vi "Golander pump(mL per s, mL per rev) old.vi"(4 "State":i16, 5 "Time":dbl format="%.2f", 6 "Sensor Values":dbl[](array[numeric]), 7 "Set Points":dbl[](array[numeric])=[12.0, 1.0, 1.0, 1.0]) -> (0 "required data":T4={"Set Point names"=["com port", "pump address", "on state (-1=all, 167= states 1, 6, 7)", "pump (mL/rev)", "flow (mL/s)"], "required number of setpoints"=5, "required number of sensors"=0, "Sensor names"=[]}, 3 "output value":dbl)   [LabVIEW 2019]
uses:
  pump 2 flows.ctl
  Pump updates.ctl
  modbusrtu/MB Serial Master Query Write Multiple Registers (poly).vi
panel:
  in  "delay before write":u32=200
  out "Pump updates":T1[](array[typedef]) {"Update Time" format="%.2f"}
  in  "Pump updates":T1 {"Update Time" format="%.2f"}
  in  "Timeout":u32=240
  in  "write interval (s)":dbl=5.0
  out "pump cmd array":T2[](array[typedef])
  out "output cluster":T3
  in  "Pump cmds":T2
  in  "error in (no error)":errorcluster
  out "VISA out":refnum<visa-resource-name>
  out "error out":errorcluster
  # "failure at 80 ms"
  # "Enter the correct information for this control code in the required data structure below. Then make the current value default by right clicking on the border of the data structure. Select \"data operations\" and then select \"make current value default\". These values will be displayed by process controller."
  # "Mode: RTU\nAddresses: 1-247 (User Defined)\nBaud Rate: 9600\nData Bits: 8\nCRC: Even Parity\nStop Bit: 1"
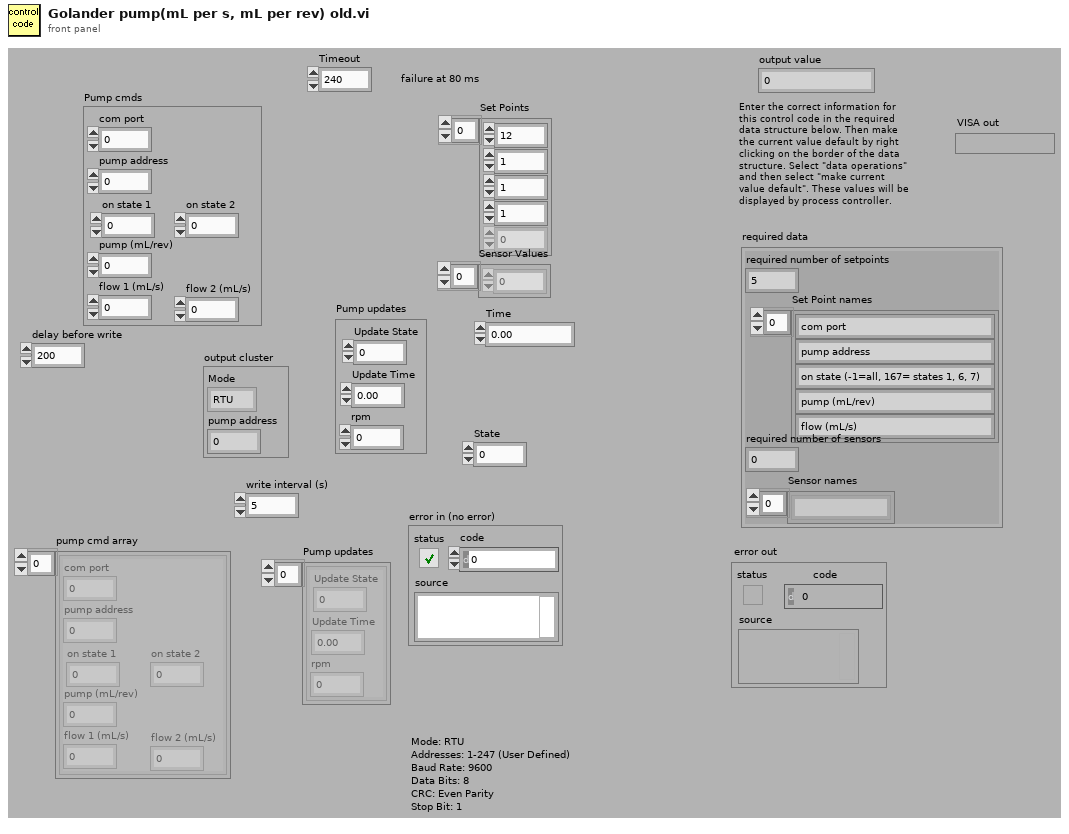
[diagram p1: front panel]
types:
  T1 = typedef "Pump updates.ctl" = cluster{"Update State":i16, "Update Time":dbl, "rpm":dbl}
  T2 = typedef "pump 2 flows.ctl" = cluster{"com port":u8, "pump address":u8, "on state 1":i32, "on state 2":i32, "pump (mL/rev)":dbl, "flow 1 (mL/s)":dbl, "flow 2 (mL/s)":dbl}
  T3 = cluster{"Mode":enum16{"RTU", "ASCII"}, "pump address":u8}
  T4 = cluster{"Set Point names":string[], "required number of setpoints":u8, "required number of sensors":u8, "Sensor names":string[]}
  T5 = cluster{"Set Points[0]":dbl, "Set Points[1]":dbl, "Set Points[2]":dbl, "Set Points[3]":dbl, "Set Points[4]":dbl}
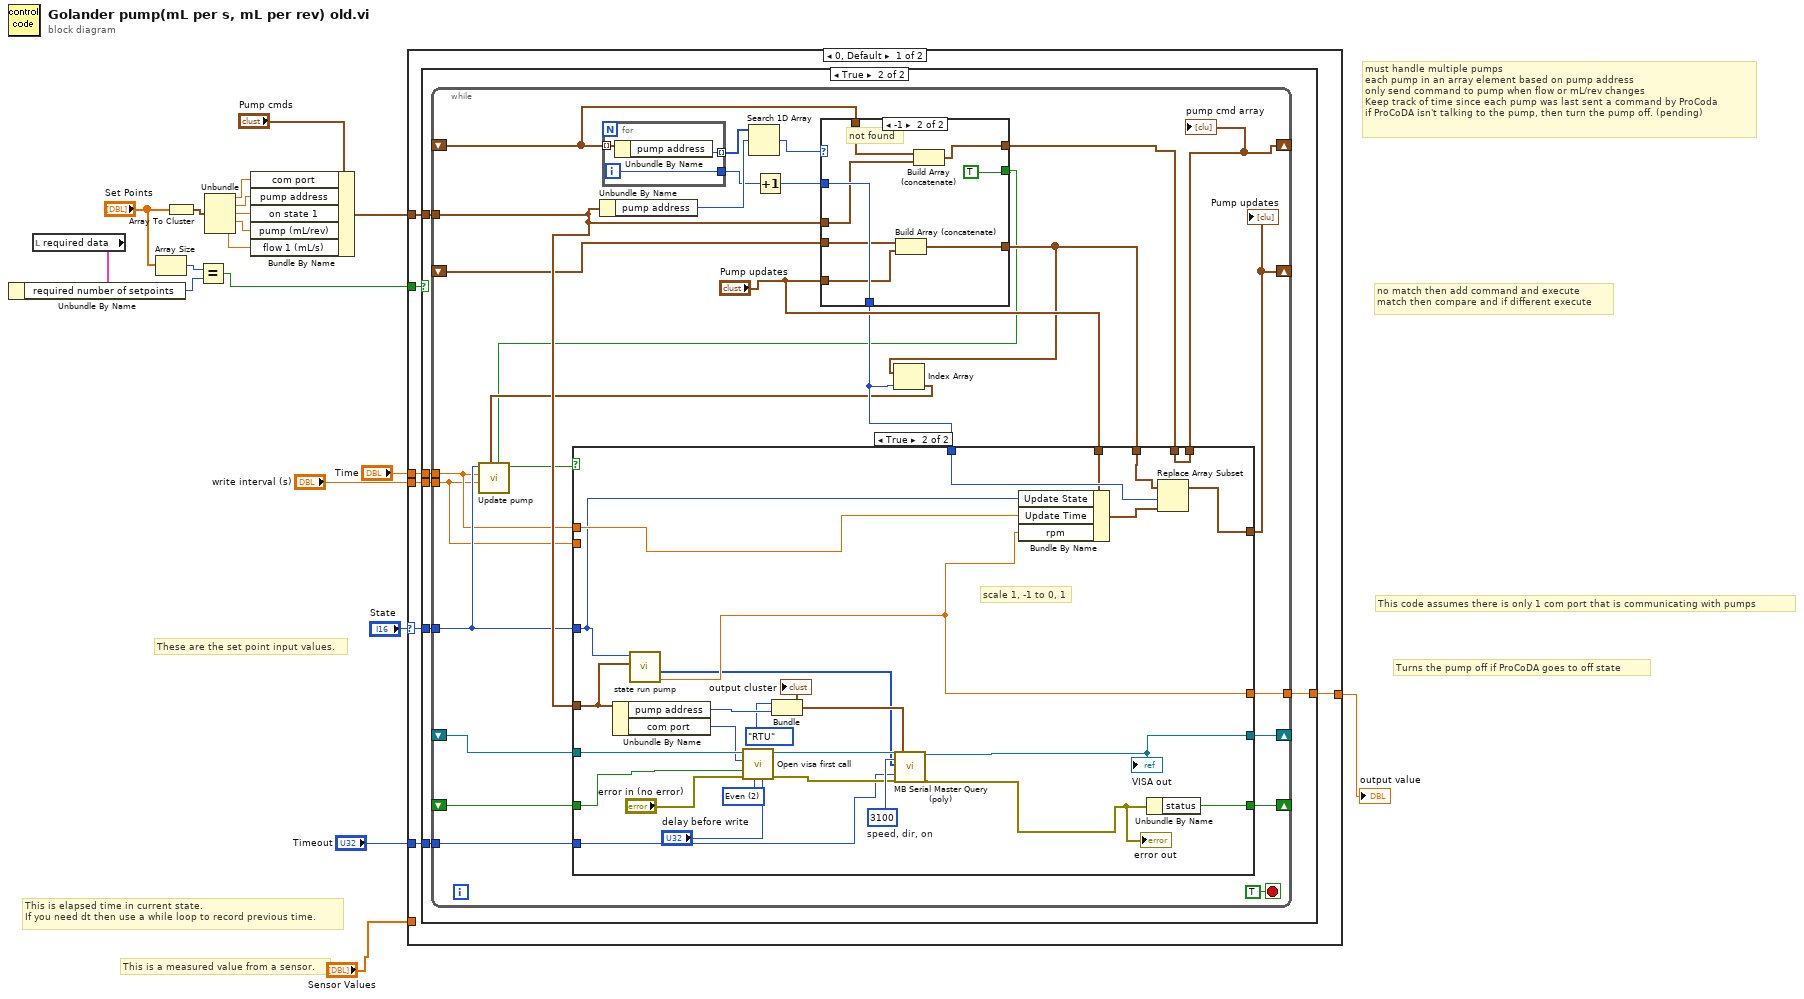
[diagram p0: block diagram]
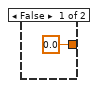
[diagram p2: hidden frame]
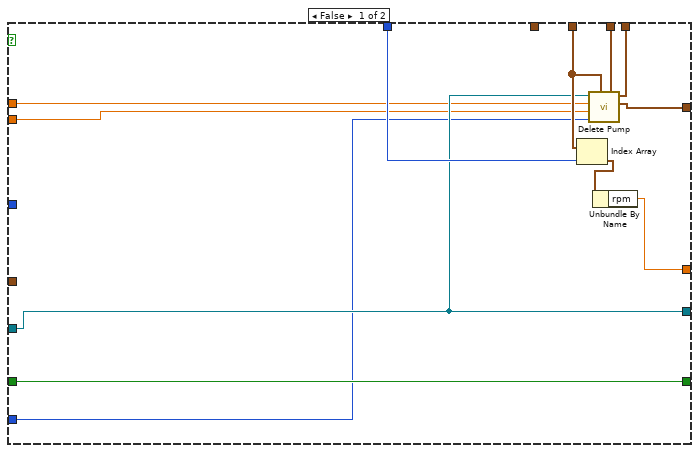
[diagram p3: hidden frame]
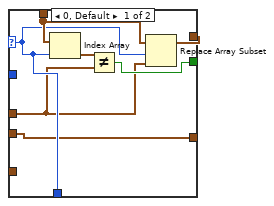
[diagram p4: hidden frame]
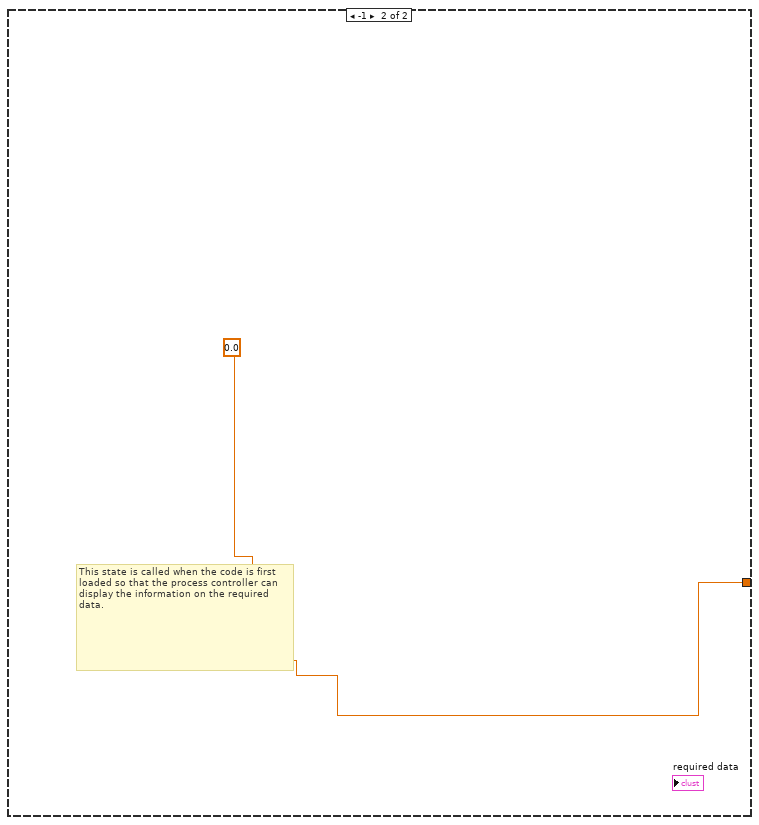
[diagram p5: hidden frame]
diagram:
  # "Turns the pump off if ProCoDA goes to off state"
  # "This code assumes there is only 1 com port that is communicating with pumps"
  # "no match then add command and execute\nmatch then compare and if different execute"
  # "must handle multiple pumps\neach pump in an array element based on pump address\nonly send command to pump when flow or mL/rev changes\nKeep track of time since each pump was last sent a command by ProCoda\nif ProCoDA isn't talking to the pump, then turn the pump off. (pending)"
  # "These are the set point input values."
  # "This is a measured value from a sensor."
  # "This is elapsed time in current state.\nIf you need dt then use a while loop to record previous time."
  n1 = local read "required data"() -> (w3:T4)
  n2 = Unbundle By Name(w3) -> ("required number of setpoints"=w2:u8)
  n3 = Array Size(array="Set Points") -> (size(s)=w5:i32)
  n4 = Array To Cluster(array="Set Points") -> (cluster=w16:T5)
  n5 = Equal?(x=w5, y=w2) -> (x = y?=w1:bool)
  n6 = Unbundle(w16) -> ("Set Points[0]"=w13:dbl, "Set Points[1]"=w17:dbl, "Set Points[2]"=w8:dbl, "Set Points[3]"=w10:dbl, "Set Points[4]"=w9:dbl)
  n7 = Bundle By Name(cluster="Pump cmds", "com port"=w13, "pump address"=w17, "on state 1"=w8, "pump (mL/rev)"=w10, "flow 1 (mL/s)"=w9) -> (w15:T2)
  n8 = case shown="0, Default" "State" {
    selector: "State" -> [w24 _]
    tunnel: [w25 0.0 ("fraction on")] -> w12
    tunnel: w15 -> [w26 _]
    tunnel: "Sensor Values" -> [_ _]
    tunnel: "Time" -> [w23 _]
    tunnel: "write interval (s)" -> [w22 _]
    tunnel: "Timeout" -> [w21 _]
    tunnel: w1 -> [w20 _]
    frame 0, Default {
      n9 = case shown="True" w20 {
        tunnel: w26 -> [_ w33]
        tunnel: [0.0 ("rpm") w32] -> w25
        tunnel: w24 -> [_ w31]
        tunnel: w23 -> [_ w30]
        tunnel: w22 -> [_ w29]
        tunnel: w21 -> [_ w28]
        frame False {
        }
        frame True {
          n10 = while {
            shift-right: [w56] -> _
            shift-left: _ -> [w59]
            tunnel: w33 -> [w48]
            shift-right: [w57] -> _
            shift-left: _ -> [w58]
            shift-right: [w35] -> _
            shift-left: _ -> [w51]
            tunnel: w31 -> [w42]
            tunnel: w30 -> [w41]
            shift-right: [w46] -> _
            shift-left: _ -> [w47]
            tunnel: w29 -> [w34]
            tunnel: [w55] -> w32
            tunnel: w28 -> [w37]
            stop <- TRUE stop-if-true
            n11 = Unbundle By Name(w48) -> ("pump address"=w53:u8)
            n12 = for {
              tunnel: [w117] -> w54 mode=indexing
              tunnel: w51 -> [w116] mode=indexing
              tunnel: [w115] -> w50
              i -> [w115]
              n13 = Unbundle By Name(w116) -> ("pump address"=w117:u8)
            }
            n14 = Search 1D Array(1D array=w54, element=w53) -> (index of element=w52:i32)  [unwired: 1 in]
            n15 = Increment(x=w50) -> (x+1=w49:i32)
            n16 = case shown="-1" w52 {
              selector: w52 -> [w102 _]
              tunnel: [w105 TRUE] -> w38
              tunnel: w51 -> [w104 w113]
              tunnel: [w103 w112] -> w36
              tunnel: w49 -> [_ w111]
              tunnel: [w102 w111] -> w44
              tunnel: w48 -> [w101 w110]
              tunnel: w47 -> [w100 w109]
              tunnel: [w100 w108] -> w43
              tunnel: "Pump updates" -> [_ w107]
              frame 0, Default {
                n17 = Index Array(array=w104, index=w102) -> (element=w106:T2)
                n18 = Not Equal?(x=w106, y=w101) -> (x != y?=w105:bool)
                n19 = Replace Array Subset(array=w104, new element=w101, index=w102) -> (w103:T2[])
              }
              frame -1 {
                # "not found"
                n20 = Build Array (concatenate)(w109, w107) -> (w108:T1[])
                n21 = Build Array (concatenate)(w113, w110) -> (w112:T2[])
              }
            }
            n22 = Index Array(array=w43, index=w44) -> (element=w40:T1)
            n23 = call "Update pump.vi"("new pump cmd"=w38, "Pump updates"=w40, "write interval (s)"=w34, "Time"=w41, "State"=w42) -> ("update"=w39:bool)  [unwired: 6 in]
            n24 = case shown="True" w39 {
              tunnel: w59 -> [w64 w98]
              tunnel: w58 -> [w72 w76]
              tunnel: [w72 w97] -> w57
              tunnel: [w64 w75] -> w56
              tunnel: [w69 w79] -> w55
              tunnel: w48 -> [_ w86]
              tunnel: w42 -> [_ w78]
              tunnel: w41 -> [w63 w83]
              tunnel: [w67 w87] -> w46
              tunnel: w43 -> [w68 w88]
              tunnel: w44 -> [w71 w84]
              tunnel: "Pump updates" -> [_ w82]
              tunnel: w37 -> [w62 w81]
              tunnel: w36 -> [w66 w80]
              tunnel: [w65 w80] -> w35
              tunnel: w34 -> [w61 _]
              frame False {
                n25 = Index Array(array=w68, index=w71) -> (element=w70:T1)
                n26 = call "Delete Pump.vi"("pump cmd array"=w66, "Pump updates"=w68, "Timeout"=w62, "write interval (s)"=w61, "Time"=w63, "VISA"=w64) -> ("Pump updates out"=w67:T1[], "pump cmd array out"=w65:T2[])  [unwired: 4 in]
                n27 = Unbundle By Name(w70) -> ("rpm"=w69:dbl)
              }
              frame True {
                w89 = u16 2 items=["None", "Odd", "Even", "Mark", "Space"] ("Parity")
                w92 = u16 3100  # speed, dir, on
                # "scale 1, -1 to 0, 1"
                n28 = Unbundle By Name(w86) -> ("pump address"=w94:u8, "com port"=w96:u8)
                n29 = call "state run pump.vi"("pump command"=w86, "State"=w78) -> ("rpm"=w79:dbl, "registers"=w77:u16[])  [unwired: 2 in, 2 out]
                n30 = call "Open visa first call.vi"("delay before write"="delay before write", "Parity"=w89, "error in (no error)"="error in (no error)", "error"=w76, "Com port"=w96, "VISA Refnum in"=w98) -> ("error out"=w91:errorcluster, "VISA Refnum out"=w95:refnum<visa-resource-name>)  [unwired: 4 in]
                n31 = Bundle("Mode"=enum16{"RTU", "ASCII"}."RTU", "pump address"=w94) -> (w90:T3)  [unwired: 1 in]
                "output cluster" <- w90
                n32 = call-poly "MB Serial Master Query (poly).vi"("VISA resource name"=w95, "Starting Address"=w92, "Registers"=w77, "Timeout"=w81, "error in"=w91, "Serial Parameters"=w90) -> ("VISA resource name out"=w75:refnum<visa-resource-name>, "error out"=w74:errorcluster)  [unwired: 11 in, 1 out]
                "VISA out" <- w75
                "error out" <- w74
                n33 = Bundle By Name(cluster=w82, "Update State"=w78, "Update Time"=w83, "rpm"=w79) -> (w85:T1)
                n34 = Unbundle By Name(w74) -> ("status"=w97:bool)
                n35 = Replace Array Subset(array=w88, new element=w85, index=w84) -> (w87:T1[])
              }
            }
            "pump cmd array" <- w35
            "Pump updates" <- w46
          }
        }
      }
    }
    frame -1 {
      # "This state is called when the code is first loaded so that the process controller can display the information on the required data."
    }
  }
  "output value" <- w12
